vi "Get page GUID.vi"(8 "error in (no error)":errorcluster, 11 "Page Name":string) -> (0 "error out":errorcluster, 3 "GUID":string)   [LabVIEW 2017, in "Data Sharing Framework System Explorer.lvlib"]
uses:
  Data Sharing Framework System Explorer.lvlib
  <vilib>/xml/Load XML File.vi
  <vilib>/xml/NI_XML.lvlib
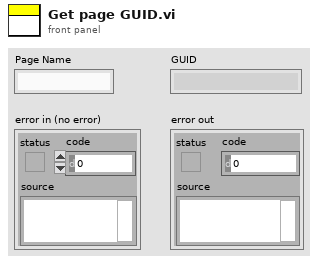
[diagram p1: front panel]
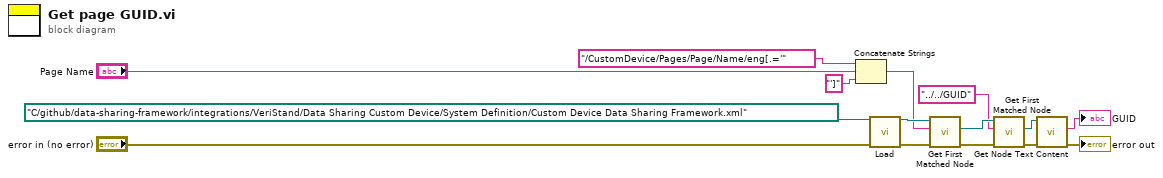
[diagram p0: block diagram]
diagram:
  n1 = Concatenate Strings("/CustomDevice/Pages/Page/Name/eng[.='" ("XPath expression"), "Page Name", "']" ("string")) -> (w6:string)
  n2 = call-poly <vilib>:"Load.vi"("path to XML document"=path "C:/github/data-sharing-framework/integrations/VeriStand/Data Sharing Custom Device/System Definition/Custom Device Data Sharing Framework.xml", "error in (no error)"="error in (no error)") -> ("DOM document out"=w14:refnum<k20>, "error out"=w5:errorcluster)  [unwired: 11 in, 1 out]
  n3 = call <vilib>:"Get First Matched Node.vi"("error in (no error)"=w5, "XPath expression"=w6, "node in"=w14) -> ("error out"=w4:errorcluster, "node result"=w13:refnum<k20>)  [unwired: 6 in, 1 out]
  n4 = call <vilib>:"Get First Matched Node.vi"("error in (no error)"=w4, "XPath expression"="../../GUID", "node in"=w13) -> ("error out"=w3:errorcluster, "node result"=w11:refnum<k20>)  [unwired: 6 in, 1 out]
  n5 = call <vilib>:"Get Node Text Content.vi"("error in (no error)"=w3, "node in"=w11) -> ("error out"=→"error out":errorcluster, "node text"=→"GUID":string)  [unwired: 7 in, 1 out]
